vi "Read DCA Pressure 2.vi"(11 "ILC in":refnum<class "ILC.lvclass">) -> (2 "DCA Pressure 2":dbl, 3 "ILC out":refnum<class "ILC.lvclass">)   [LabVIEW 2015, in "ILCCommon.lvlib" / "ILC.lvclass"]
uses:
  <userlib>/Common/ILC/ILC/ILC.lvclass
  <userlib>/Common/ILC/ILC/ILC.lvclass/ILC.ctl
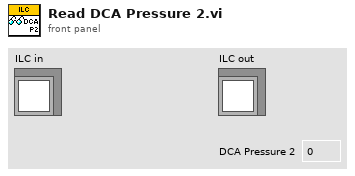
[diagram p1: front panel]
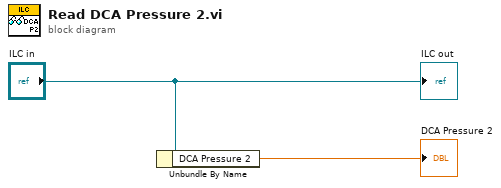
[diagram p0: block diagram]
diagram:
  n1 = Unbundle By Name("ILC in") -> ("DCA Pressure 2"=→"DCA Pressure 2":dbl)
  "ILC out" <- "ILC in"
